vi "startUp.vi"(8 "error in (no error)":errorcluster, 10 "ScriptEvent":refnum<class "ScriptEvent.lvclass">, 11 "ActionPanel in":refnum<class "ActionPanel.lvclass">) -> (0 "error out":errorcluster, 3 "ActionPanel out":refnum<class "ActionPanel.lvclass">)   [LabVIEW 2011, in "Views.lvlib" / "ScriptEditor.lvlib" / "ActionPanel.lvclass"]
uses:
  ActionPanel.lvclass
  Tools/Scripting/ScriptingEvent/ScriptEvent.lvclass
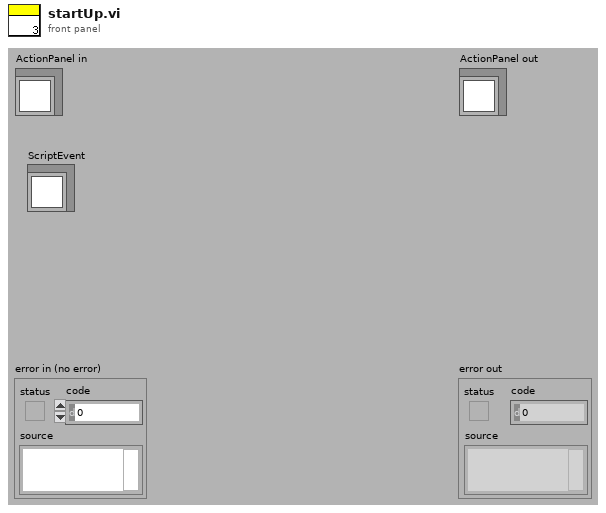
[diagram p1: front panel]
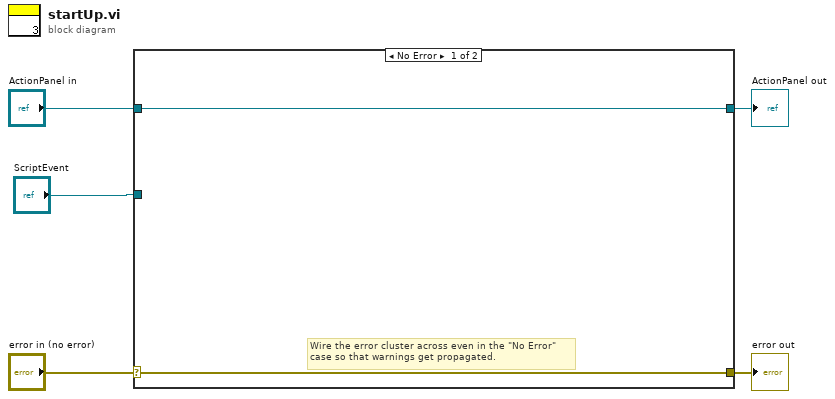
[diagram p0: block diagram]
diagram:
  n1 = case shown="No Error" "error in (no error)" {
    selector: "error in (no error)" -> [w6 w9]
    tunnel: [w6 w9] -> w4
    tunnel: [w7 w8] -> w2
    tunnel: "ActionPanel in" -> [w7 w8]
    tunnel: "ScriptEvent" -> [_ _]
    frame No Error {
      # "Wire the error cluster across even in the \"No Error\"\ncase so that warnings get propagated."
    }
    frame Error {
    }
  }
  "error out" <- w4
  "ActionPanel out" <- w2
